vi "Wax Melter.vi"() -> ()   [LabVIEW 2020]
uses:
  state.ctl
  <vilib>/DAQmx/write.llb/DAQmx Write (Digital Bool 1Line 1Point).vi
  <vilib>/DAQmx/create/channels.llb/DAQmx Create Channel (AI-Resistance).vi
  <vilib>/DAQmx/create/channels.llb/DAQmx Create Channel (DO-Digital Output).vi
  <vilib>/DAQmx/miscellaneous.llb/DAQmx Fill In Error Info.vi
panel:
  out "Heating":bool
  out "TGT Temp (F)":dbl format="%#_3g"
  out "Current State":T1=enum."Start"
  in  "Exit":bool
  in  "Start":bool
  out "ACT Temp (F)":dbl format="%#_3g"
  out "Resistance (Ohms)":dbl format="%0.2f"
  in  "Target Temperature (F)":dbl(slide) scale=0.0..300.0
  out "Waveform Chart":cluster{"Temp (F)":dbl, dbl}(graph)
  in  "Stop":bool
  out "Temperature":dbl(knob) scale=0.0..300.0
  out "Tgt Temp Gauge":dbl(knob) scale=0.3..300.0
  # "Candlescience Wax Melter"
  # "Resistance (Ohms)"
  # "Temperature (F)"
  # "Samples"
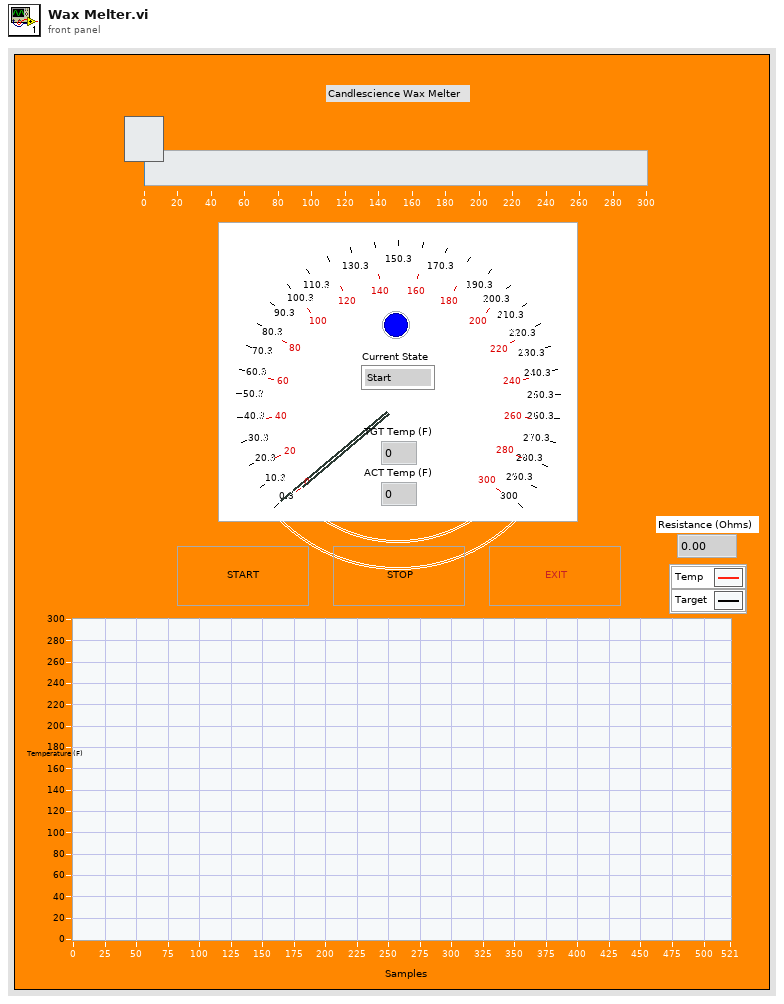
[diagram p1: front panel]
types:
  T1 = typedef "state.ctl" = enum16{"Cooling", "Heating", "Start", "Stop", "Idle", "Init"}
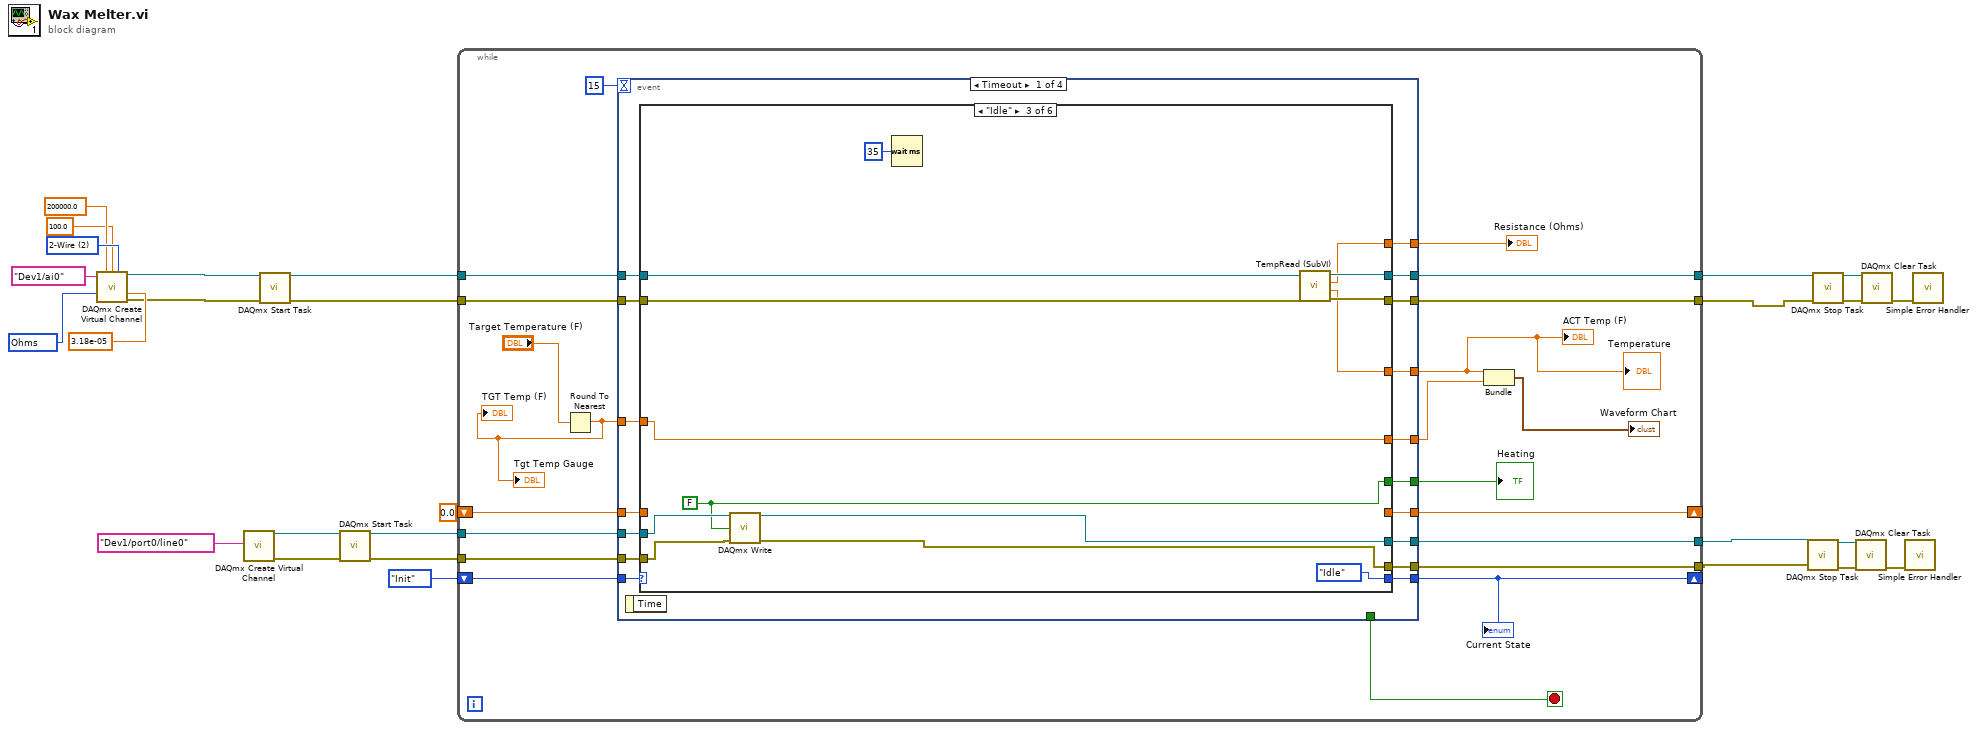
[diagram p0: block diagram]
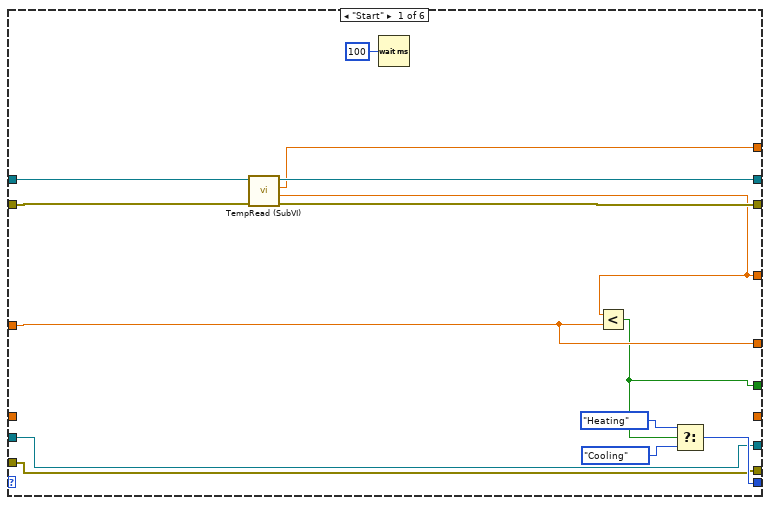
[diagram p2: hidden frame]
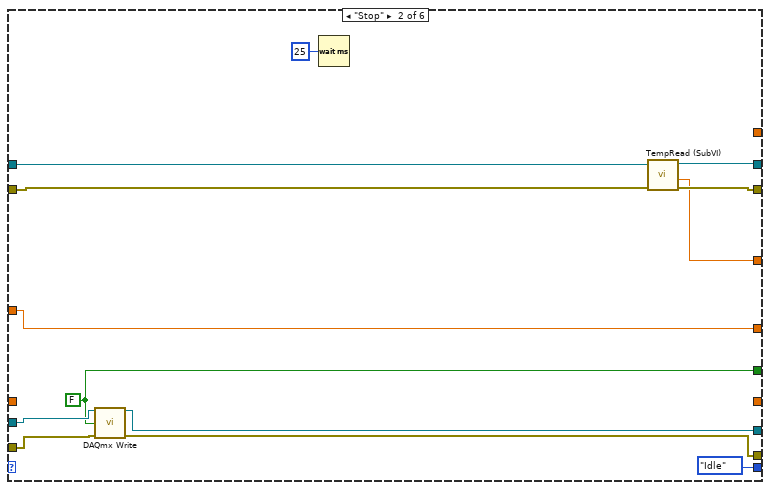
[diagram p3: hidden frame]
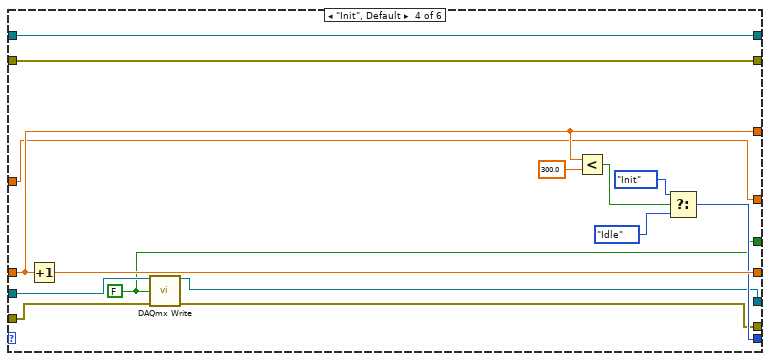
[diagram p4: hidden frame]
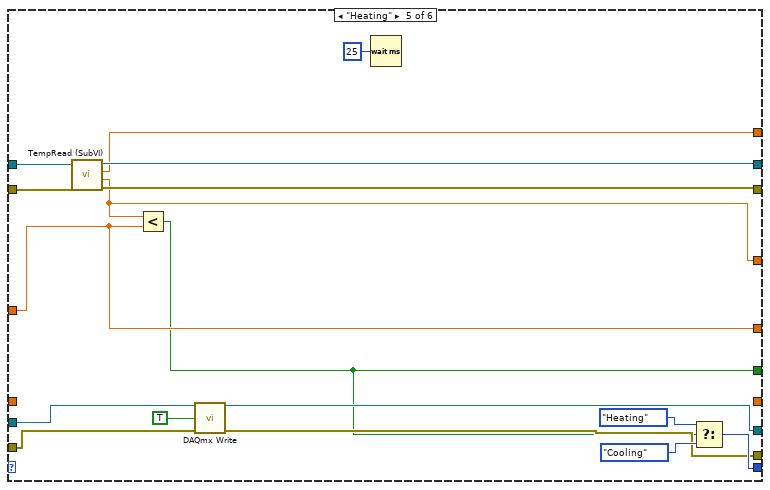
[diagram p5: hidden frame]
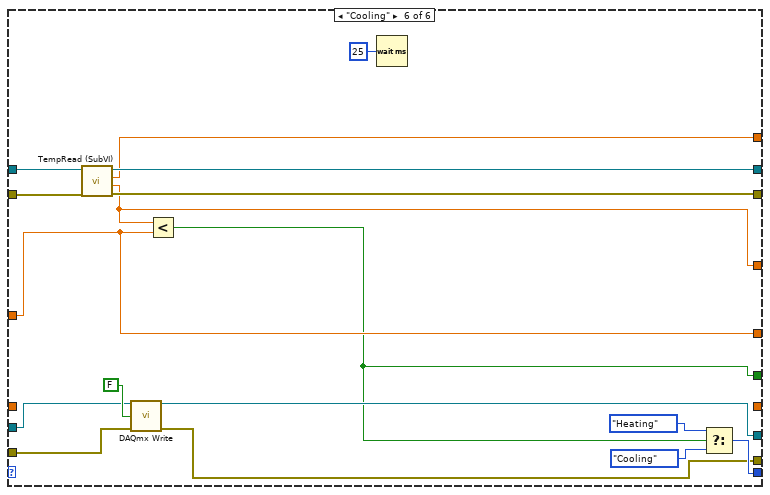
[diagram p6: hidden frame]
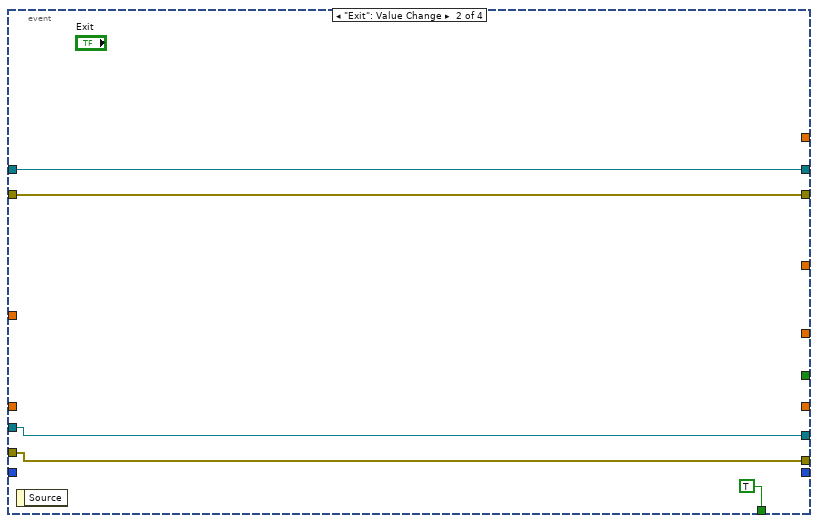
[diagram p7: hidden frame]
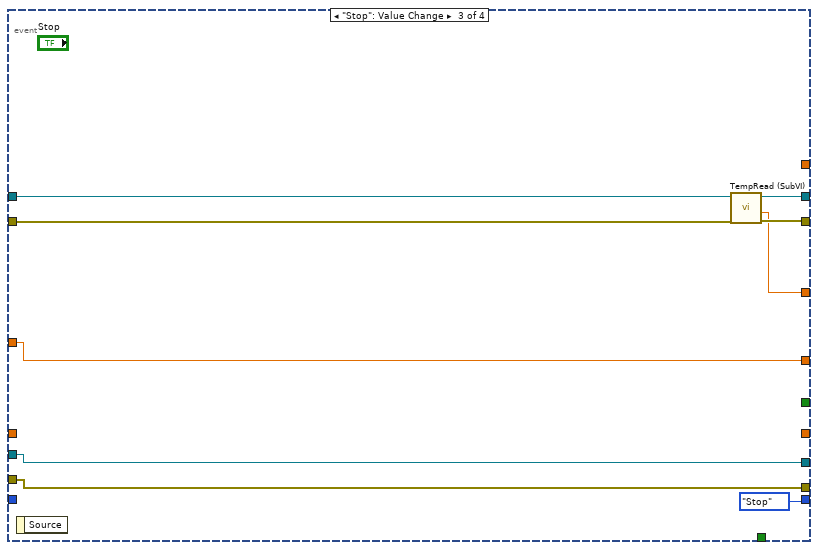
[diagram p8: hidden frame]
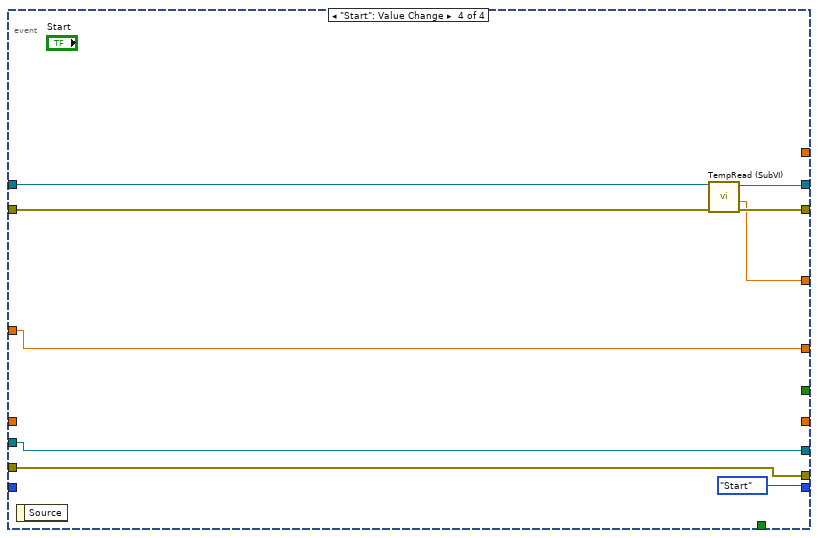
[diagram p9: hidden frame]
diagram:
  w20 = 10384 items=["Ohms"=10384, "From Custom Scale"=10065] ("units")
  w21 = 2 items=["2-Wire"=2, "3-Wire"=3, "4-Wire"=4] ("resistance configuration")
  n1 = call-poly <vilib>:"DAQmx Create Virtual Channel.vi"("maximum value"=200000.0, "minimum value"=100.0, "resistance configuration"=w21, "physical channels"=tag "Dev1/ai0", "units"=w20, "current excitation value"=3.18e-05) -> ("task out"=w14:refnum<k21>, "error out"=w13:errorcluster)  [unwired: 8 in]
  n2 = call-poly <vilib>:"DAQmx Create Virtual Channel.vi"("lines"=tag "Dev1/port0/line0") -> ("task out"=w12:refnum<k21>, "error out"=w11:errorcluster)  [unwired: 13 in]
  n3 = call <vilib>:"DAQmx Start Task.vi"("task/channels in"=w14, "error in"=w13) -> ("task out"=w27:refnum<k21>, "error out"=w26:errorcluster)  [unwired: 12 in]
  n4 = call <vilib>:"DAQmx Start Task.vi"("task/channels in"=w12, "error in"=w11) -> ("task out"=w10:refnum<k21>, "error out"=w9:errorcluster)  [unwired: 12 in]
  n5 = while {
    tunnel: w27 -> [w48]
    tunnel: w26 -> [w47]
    tunnel: [w46] -> w1
    tunnel: [w45] -> w2
    shift-right: [w43] -> _
    shift-left: state."Init" -> [w44]
    shift-right: [w39] -> _
    shift-left: 0.0 -> [w40]
    tunnel: w10 -> [w32]
    tunnel: w9 -> [w31]
    tunnel: [w30] -> w4
    tunnel: [w29] -> w3
    stop <- w41 stop-if-true
    n6 = Round To Nearest(number="Target Temperature (F)") -> (nearest integer value=w37:dbl)
    "Tgt Temp Gauge" <- w37
    "TGT Temp (F)" <- w37
    n7 = event shown="[0] Timeout" {
      selector: _ -> [_ _ _ _]
      dyn-events: _ -> [_ _ _ _]
      timeout: 15 -> [_ _ _ _]
      tunnel: w48 -> [w65 w159 w165 w174]
      tunnel: w47 -> [w64 w158 w163 w172]
      tunnel: [w63 w159 w164 w173] -> w46
      tunnel: [w62 w158 w162 w171] -> w45
      tunnel: w44 -> [w61 _ _ _]
      tunnel: [w60 _ state."Stop" state."Start"] -> w43
      tunnel: [w59 _ w161 w170] -> w34
      tunnel: [_ TRUE _ _] -> w41
      tunnel: w40 -> [w58 _ _ _]
      tunnel: [w57 _ _ _] -> w39
      tunnel: w37 -> [w56 _ w166 w175]
      tunnel: [w55 _ w166 w175] -> w36
      tunnel: [w54 _ _ _] -> w33
      tunnel: w32 -> [w53 w157 w168 w177]
      tunnel: w31 -> [w52 w156 w167 w176]
      tunnel: [w51 w157 w168 w177] -> w30
      tunnel: [w50 w156 w167 w176] -> w29
      tunnel: [w49 _ _ _] -> w28
      event Timeout {
        n8 = event-data() -> ()  [unwired: 1 in, 1 out]
        n9 = case shown="\"Idle\"" w61 {
          tunnel: w65 -> [w78 w84 w100 w121 w138 w153]
          tunnel: w64 -> [w77 w83 w99 w120 w137 w152]
          tunnel: [w76 w82 w103 w121 w136 w151] -> w63
          tunnel: [w75 w81 w102 w120 w135 w150] -> w62
          tunnel: [w72 state."Idle" state."Idle" w113 w132 w149] -> w60
          tunnel: [w74 w80 w101 w118 w131 w148] -> w59
          tunnel: w58 -> [_ _ _ w118 _ _]
          tunnel: [_ _ _ w119 _ _] -> w57
          tunnel: w56 -> [w70 w90 w104 w112 w129 w146]
          tunnel: [w70 w90 w104 w112 w129 w146] -> w55
          tunnel: [w69 _ w98 _ w128 w145] -> w54
          tunnel: w53 -> [w68 w89 w97 w111 w127 w143]
          tunnel: w52 -> [w67 w87 w96 w110 w126 w142]
          tunnel: [w68 w88 w95 w109 w125 w141] -> w51
          tunnel: [w67 w86 w94 w108 w124 w140] -> w50
          tunnel: [w66 w85 w93 w107 w122 w139] -> w49
          frame "Start" {
            n10 = call "TempRead (SubVI).vi"("error in (no error)"=w77, "Refnum in"=w78) -> ("error out"=w75:errorcluster, "Temp (F)"=w74:dbl, "Resistance"=w69:dbl, "Refnum out"=w76:refnum<k21>)  [unwired: 6 in]
            n11 = Wait (ms)(milliseconds to wait=u32 100) -> ()  [unwired: 1 out]
            n12 = Less?(x=w74, y=w70) -> (x < y?=w66:bool)
            n13 = Select(t=state."Heating", s=w66, f=state."Cooling") -> (s? t:f=w72:T1)
          }
          frame "Stop" {
            w85 = FALSE ("data")
            n14 = call-poly <vilib>:"DAQmx Write.vi"("task/channels in"=w89, "data"=w85, "error in"=w87) -> ("task out"=w88:refnum<k21>, "error out"=w86:errorcluster)  [unwired: 10 in, 1 out]
            n15 = Wait (ms)(milliseconds to wait=u32 25) -> ()  [unwired: 1 out]
            n16 = call "TempRead (SubVI).vi"("error in (no error)"=w83, "Refnum in"=w84) -> ("error out"=w81:errorcluster, "Temp (F)"=w80:dbl, "Refnum out"=w82:refnum<k21>)  [unwired: 6 in, 1 out]
          }
          frame "Idle" {
            w93 = FALSE ("data")
            n17 = call-poly <vilib>:"DAQmx Write.vi"("task/channels in"=w97, "data"=w93, "error in"=w96) -> ("task out"=w95:refnum<k21>, "error out"=w94:errorcluster)  [unwired: 10 in, 1 out]
            n18 = Wait (ms)(milliseconds to wait=u32 35) -> ()  [unwired: 1 out]
            n19 = call "TempRead (SubVI).vi"("error in (no error)"=w99, "Refnum in"=w100) -> ("error out"=w102:errorcluster, "Temp (F)"=w101:dbl, "Resistance"=w98:dbl, "Refnum out"=w103:refnum<k21>)  [unwired: 6 in]
          }
          frame "Init", Default {
            w107 = FALSE ("data")
            n20 = Increment(x=w118) -> (x+1=w119:dbl)
            n21 = call-poly <vilib>:"DAQmx Write.vi"("task/channels in"=w111, "data"=w107, "error in"=w110) -> ("task out"=w109:refnum<k21>, "error out"=w108:errorcluster)  [unwired: 10 in, 1 out]
            n22 = Less?(x=w118, y=300.0) -> (x < y?=w116:bool)
            n23 = Select(t=state."Init", s=w116, f=state."Idle") -> (s? t:f=w113:T1)
          }
          frame "Heating" {
            n24 = call "TempRead (SubVI).vi"("error in (no error)"=w137, "Refnum in"=w138) -> ("error out"=w135:errorcluster, "Temp (F)"=w131:dbl, "Resistance"=w128:dbl, "Refnum out"=w136:refnum<k21>)  [unwired: 6 in]
            n25 = Less?(x=w131, y=w129) -> (x < y?=w122:bool)
            n26 = call-poly <vilib>:"DAQmx Write.vi"("task/channels in"=w127, "data"=TRUE, "error in"=w126) -> ("task out"=w125:refnum<k21>, "error out"=w124:errorcluster)  [unwired: 10 in, 1 out]
            n27 = Wait (ms)(milliseconds to wait=u32 25) -> ()  [unwired: 1 out]
            n28 = Select(t=state."Heating", s=w122, f=state."Cooling") -> (s? t:f=w132:T1)
          }
          frame "Cooling" {
            n29 = call "TempRead (SubVI).vi"("error in (no error)"=w152, "Refnum in"=w153) -> ("error out"=w150:errorcluster, "Temp (F)"=w148:dbl, "Resistance"=w145:dbl, "Refnum out"=w151:refnum<k21>)  [unwired: 6 in]
            n30 = call-poly <vilib>:"DAQmx Write.vi"("task/channels in"=w143, "data"=FALSE, "error in"=w142) -> ("task out"=w141:refnum<k21>, "error out"=w140:errorcluster)  [unwired: 10 in, 1 out]
            n31 = Less?(x=w148, y=w146) -> (x < y?=w139:bool)
            n32 = Wait (ms)(milliseconds to wait=u32 25) -> ()  [unwired: 1 out]
            n33 = Select(t=state."Heating", s=w139, f=state."Cooling") -> (s? t:f=w149:T1)
          }
        }
      }
      event "Exit": Value Change {
        n34 = event-data() -> ()  [unwired: 1 in, 1 out]
      }
      event "Stop": Value Change {
        n35 = event-data() -> ()  [unwired: 1 in, 1 out]
        n36 = call "TempRead (SubVI).vi"("error in (no error)"=w163, "Refnum in"=w165) -> ("error out"=w162:errorcluster, "Temp (F)"=w161:dbl, "Refnum out"=w164:refnum<k21>)  [unwired: 6 in, 1 out]
      }
      event "Start": Value Change {
        n37 = event-data() -> ()  [unwired: 1 in, 1 out]
        n38 = call "TempRead (SubVI).vi"("error in (no error)"=w172, "Refnum in"=w174) -> ("error out"=w171:errorcluster, "Temp (F)"=w170:dbl, "Refnum out"=w173:refnum<k21>)  [unwired: 6 in, 1 out]
      }
    }
    "Temperature" <- w34
    "ACT Temp (F)" <- w34
    "Current State" <- w43
    "Resistance (Ohms)" <- w33
    "Heating" <- w28
    n39 = Bundle("Temp (F)"=w34, w36) -> (→"Waveform Chart":cluster{"Temp (F)":dbl, dbl})  [unwired: 1 in]
  }
  n40 = call <vilib>:"DAQmx Stop Task.vi"("task/channels in"=w4, "error in"=w3) -> ("task out"=w5:refnum<k21>, "error out"=w8:errorcluster)  [unwired: 12 in]
  n41 = call <vilib>:"DAQmx Stop Task.vi"("task/channels in"=w1, "error in"=w2) -> ("task out"=w24:refnum<k21>, "error out"=w25:errorcluster)  [unwired: 12 in]
  n42 = call <vilib>:"DAQmx Clear Task.vi"("task in"=w5, "error in"=w8) -> ("error out"=w7:errorcluster)  [unwired: 13 in]
  n43 = call <vilib>:"DAQmx Clear Task.vi"("task in"=w24, "error in"=w25) -> ("error out"=w23:errorcluster)  [unwired: 13 in]
  n44 = call <vilib>:"Simple Error Handler.vi"("error in (no error)"=w7) -> ()  [unwired: 4 in, 5 out]
  n45 = call <vilib>:"Simple Error Handler.vi"("error in (no error)"=w23) -> ()  [unwired: 4 in, 5 out]
